vi "DC miliCurrent Configuration.vi"(8 "error in (no error)":errorcluster, 10 "Mili Current Range":T1, 11 "VISA resource name":refnum<visa-resource-name>) -> (0 "error out":errorcluster, 3 "VISA resource name out":refnum<visa-resource-name>)   [LabVIEW 2024, in "U1250 Series Digital Multimeter.lvlib"]
uses:
  <instrlib>/U1250 Series Multimeter Device Driver/U1250 Series Digital Multimeter.lvlib
  <instrlib>/U1250 Series Multimeter Device Driver/Controls/Mili Current Range.ctl
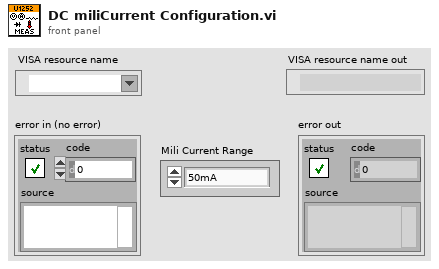
[diagram p1: front panel]
types:
  T1 = typedef "U1250 Series Digital Multimeter.lvlib/Mili Current Range.ctl" = enum16{"50mA", "500mA", "Auto"}
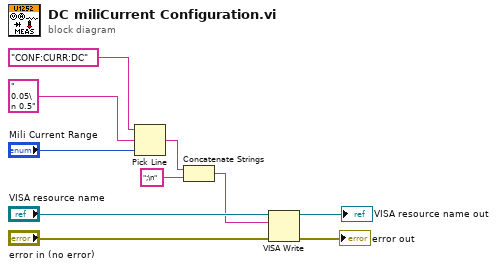
[diagram p0: block diagram]
diagram:
  n1 = Pick Line(string ("")="CONF:CURR:DC", multi-line string=" 0.05\n 0.5", line index="Mili Current Range") -> (output string=w4:string)
  n2 = Concatenate Strings(w4, ";\n" ("string")) -> (w2:string)
  n3 = VISA Write(VISA resource name="VISA resource name", write buffer=w2, error in (no error)="error in (no error)") -> (VISA resource name out=→"VISA resource name out":refnum<visa-resource-name>, error out=→"error out":errorcluster)  [unwired: 1 out]
